vi "Load_STS_param_options_SubVI.vi"(10 "STSparam.txt location":path, 11 "Array in":refnum<vi>) -> (0 "error out":errorcluster, 3 "Array":string[](array[string]))   [LabVIEW 2014]
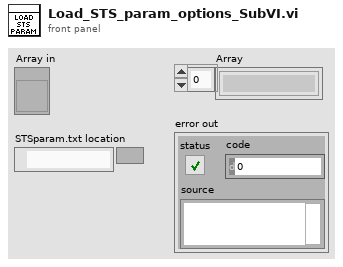
[diagram p1: front panel]
types:
  T1 = cluster{"Amplitude (mod. signal unit)":sgl, "Lockin on/off status":bool, "Advanced options":cluster{"Z-Controller Hold":bool, "Record final Z":bool, "Reset Bias":bool}, "Backward sweep":bool, "Number of points":i32, "Channels":string[], "Parameters":string[], "Fixed parameters":string[], "Multiple sweeps configuration":cluster{"Number of Sweeps":i32, "Save all":bool}, "Initialization":cluster{"Z averaging time (s)":sgl, "Z offset (m)":sgl, "Initial settling time (s)":sgl}, "Sweep Timing":cluster{"Max. slew rate (V/s)":sgl, "Settling time (s)":sgl, "Integration time (s)":sgl}, "End of Sweep":cluster{"End settling time (s)":sgl, "Z control time (s)":sgl}, "Start value (V)":sgl, "End value (V)":sgl, "Channels 2":i32[], "Name":string}[]
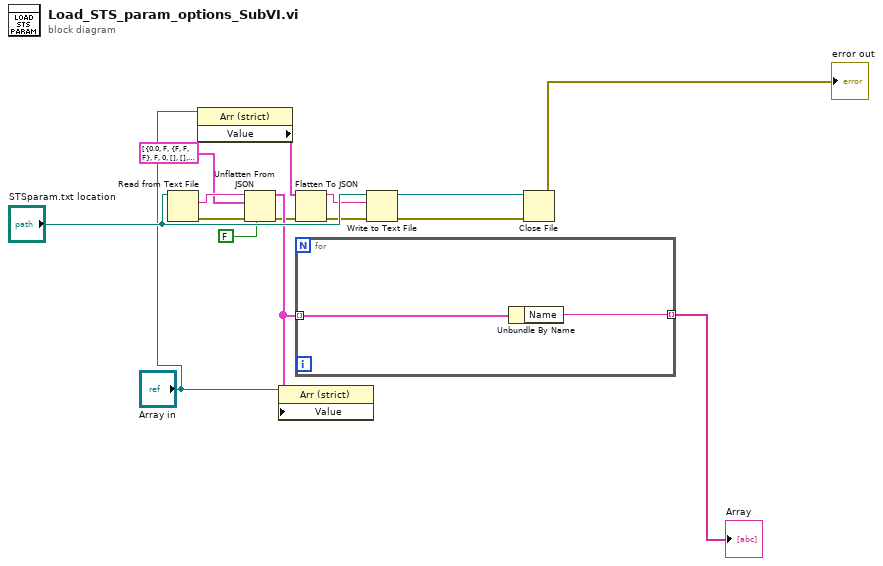
[diagram p0: block diagram]
diagram:
  n1 = Read from Text File(file (use dialog)="STSparam.txt location") -> (text=w8:string, error out=w9:errorcluster)  [unwired: 3 in, 2 out]
  n2 = property class="Arr (strict)"(reference="Array in") -> ("Value"=w13:T1)  [unwired: 1 in, 2 out]
  n3 = Unflatten From JSON(JSON string=w8, type and defaults=T1 [{"Amplitude (mod. signal unit)"=0.0, "Lockin on/off status"=FALSE, "Advanced options"={"Z-Controller Hold"=FALSE, "Record final Z"=FALSE, "Reset Bias"=FALSE}, "Backward sweep"=FALSE, "Number of points"=0, "Channels"=[], "Parameters"=[], "Fixed parameters"=[], "Multiple sweeps configuration"={"Number of Sweeps"=0, "Save all"=FALSE}, "Initialization"={"Z averaging time (s)"=0.0, "Z offset (m)"=0.0, "Initial settling time (s)"=0.0}, "Sweep Timing"={"Max. slew rate (V/s)"=0.0, "Settling time (s)"=0.0, "Integration time (s)"=0.0}, "End of Sweep"={"End settling time (s)"=0.0, "Z control time (s)"=0.0}, "Start value (V)"=0.0, "End value (V)"=0.0, "Channels 2"=[], "Name"=""}, {"Amplitude (mod. signal unit)"=0.0015, "Lockin on/off status"=FALSE, "Advanced options"={"Z-Controller Hold"=TRUE, "Record final Z"=FALSE, "Reset Bias"=TRUE}, "Backward sweep"=TRUE, "Number of points"=128, "Channels"=["Current (A)", "LI Demod 1 X (A)", "LI Demod 1 Y (A)", "LI Demod 2 X (A)", "LI Demod 2 Y (A)"], "Parameters"=["X (m)", "Y (m)", "Z (m)", "Z offset (m)", "Settling time (s)", "Integration time (s)", "Z-Ctrl hold", "Final Z (m)"], "Fixed parameters"=["Sweep Start", "Sweep End"], "Multiple sweeps configuration"={"Number of Sweeps"=100, "Save all"=FALSE}, "Initialization"={"Z averaging time (s)"=0.001, "Z offset (m)"=0.0, "Initial settling time (s)"=5e-05}, "Sweep Timing"={"Max. slew rate (V/s)"=inf, "Settling time (s)"=0.001, "Integration time (s)"=0.0005}, "End of Sweep"={"End settling time (s)"=5e-05, "Z control time (s)"=0.0}, "Start value (V)"=-0.02, "End value (V)"=0.02, "Channels 2"=[0, 20, 21, 22, 23], "Name"="Numerical_-20mV->20mV"}] ("data"), default null elements? (F)=FALSE, error in (no error)=w9) -> (value=w6:T1, error out=w2:errorcluster)  [unwired: 3 in]
  n4 = property class="Arr (strict)"(reference="Array in", "Value"=w6) -> ()  [unwired: 1 in, 2 out]
  n5 = Flatten To JSON(anything=w13, error in (no error)=w2) -> (JSON string=w10:string, 11:w14:errorcluster)  [unwired: 1 in]
  n6 = for {
    tunnel: w6 -> [w17] mode=indexing
    tunnel: [w16] -> w5 mode=indexing
    n7 = Unbundle By Name(w17) -> ("Name"=w16:string)
  }
  "Array" <- w5
  n8 = Write to Text File(file (use dialog)="STSparam.txt location", text=w10, error in=w14) -> (refnum out=w11:refnum<file>, error out=w12:errorcluster)  [unwired: 1 in, 1 out]
  n9 = Close File(refnum=w11, error in=w12) -> (error out=→"error out":errorcluster)  [unwired: 1 out]
